vi "factorial.vi"() -> ()   [LabVIEW 2018]
panel:
  out "Factorial":dbl
  in  "Number":dbl
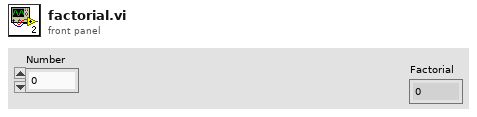
[diagram p1: front panel]
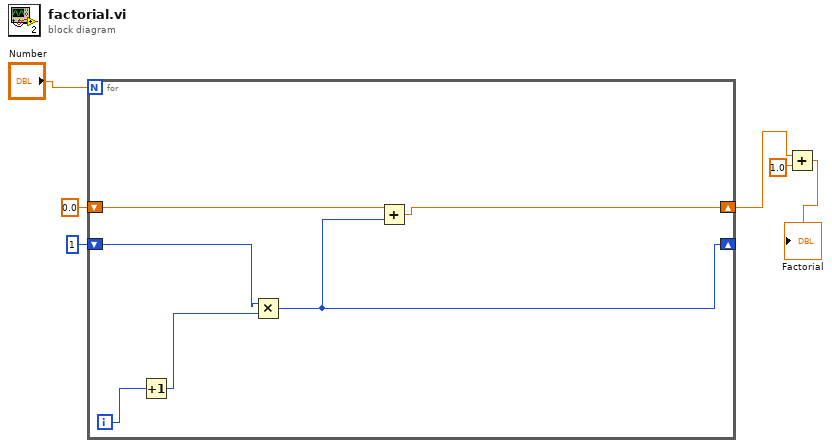
[diagram p0: block diagram]
diagram:
  n1 = for {
    N: "Number" -> [_]
    shift-right: [w10] -> w2
    shift-left: 0.0 -> [w7]
    shift-right: [w8] -> _
    shift-left: 1 -> [w9]
    i -> [w12]
    n2 = Increment(x=w12) -> (x+1=w11:i32)
    n3 = Multiply(x=w9, y=w11) -> (x*y=w8:i32)
    n4 = Add(x=w7, y=w8) -> (x+y=w10:dbl)
  }
  n5 = Add(x=w2, y=1.0) -> (x+y=→"Factorial":dbl)
